vi "Understanding Case Structure.vi"() -> ()   [LabVIEW 2026]
panel:
  in  "Boolean":bool
  out "Fahrenheit":dbl(slide) scale=0.0..500.0
  in  "Celsius":dbl(slide) scale=0.0..100.0
  out "Fahrenheit Indicator":dbl
  out "Celsius Indicator":dbl
  in  "stop":bool
  # "Understanding Case Structure"
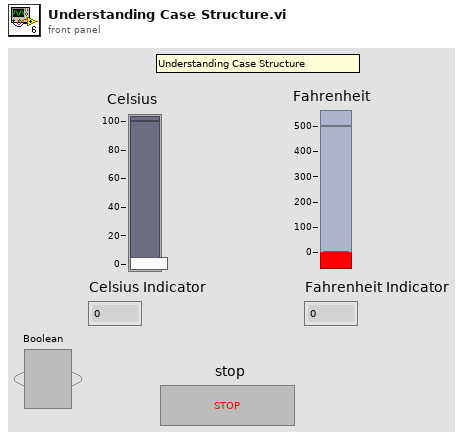
[diagram p1: front panel]
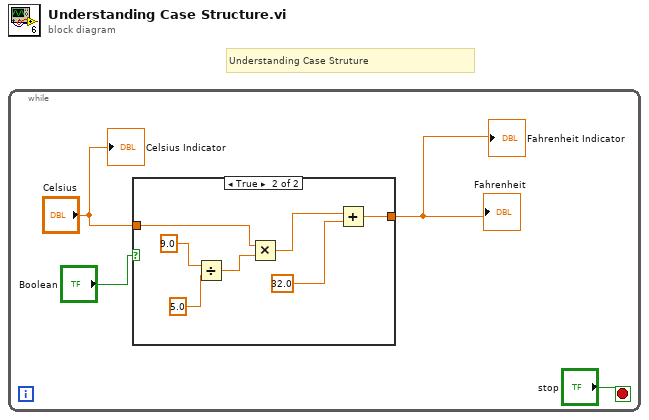
[diagram p0: block diagram]
diagram:
  # "Understanding Case Struture"
  n1 = while {
    stop <- "stop" stop-if-true
    n2 = case shown="True" "Boolean" {
      tunnel: [w5 w7] -> w4
      tunnel: "Celsius" -> [w5 w6]
      frame False {
      }
      frame True {
        n3 = Divide(x=9.0, y=5.0) -> (x/y=w11:dbl)
        n4 = Multiply(x=w6, y=w11) -> (x*y=w10:dbl)
        n5 = Add(x=w10, y=32.0) -> (x+y=w7:dbl)
      }
    }
    "Fahrenheit" <- w4
    "Fahrenheit Indicator" <- w4
    "Celsius Indicator" <- "Celsius"
  }
